vi "Is EXE.vi"(8 "Error In":errorcluster) -> (0 "Error Out":errorcluster, 2 "Application:Kind":T1(ring), 3 "T = is EXE":bool)   [LabVIEW 2016, in "Error Manager.lvlib"]
uses:
  Error Manager.lvlib
panel:
  # "Input\nInputs to the VI"
  # "Development\nControls or indicators that are useful for development or testing, but which are not outputs of the VI."
  # "Output\nOutputs of the VI"
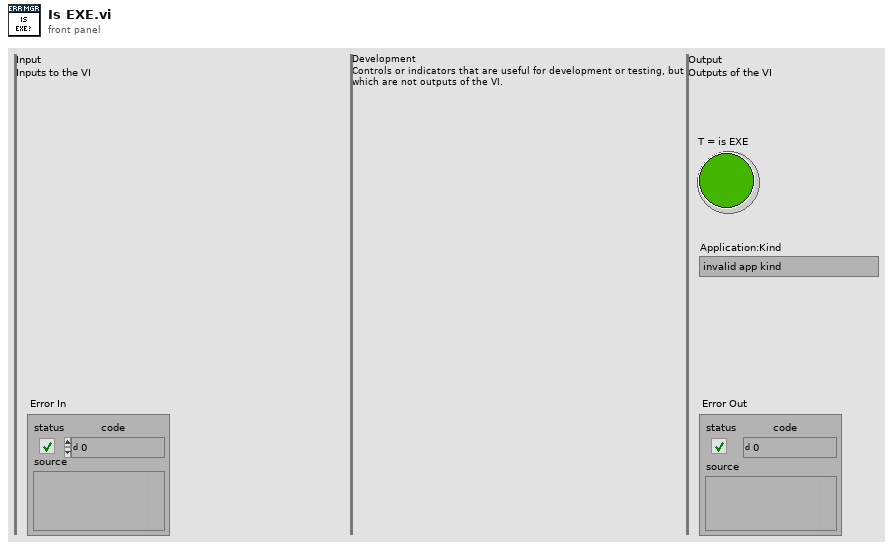
[diagram p1: front panel]
types:
  T1 = enum32{"invalid app kind", "Development System", "Run Time System", "Student Edition", "Embedded LabVIEW", "Evaluation", "Custom"}
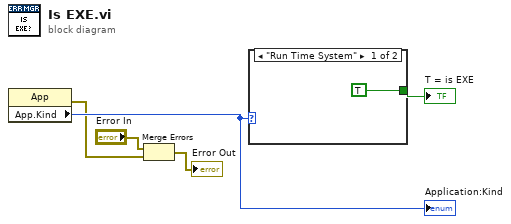
[diagram p0: block diagram]
diagram:
  n1 = property class="App"() -> (error out=w3:errorcluster, "App.Kind"=w5:T1)  [unwired: 2 in, 1 out]
  "Application:Kind" <- w5
  n2 = Merge Errors("Error In", w3) -> (→"Error Out":errorcluster)
  n3 = case shown="\"Run Time System\"" w5 {
    tunnel: [TRUE _] -> w1
    frame "Run Time System" {
    }
    frame Default {
    }
  }
  "T = is EXE" <- w1
